vi "haltnow.vi"() -> ()   [LabVIEW 2020]
panel:
  out "HaltNow":bool
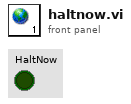
[diagram p1: front panel]
diagram:
